vi "9941 Msg Received Event is null--error.vi"(8 "error in":errorcluster) -> (0 "error out":errorcluster, 2 "Error Code":i32)   [LabVIEW 2020, in "CANopen.lvlib" / "Response Matcher.lvclass"]
uses:
  Response Matcher.lvclass
  Response Matcher.lvclass/Response Matcher.ctl
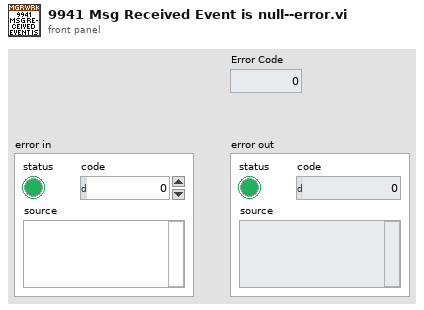
[diagram p1: front panel]
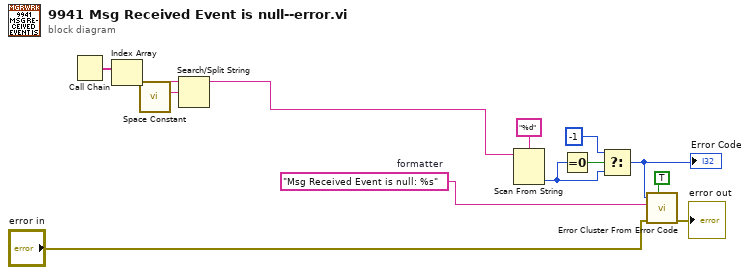
[diagram p0: block diagram]
diagram:
  w11 = "Msg Received Event is null: %s"  # formatter
  n1 = Call Chain() -> (call chain=w5:string[])
  n2 = Index Array(array=w5) -> (element=w9:string)  [unwired: 1 in]
  n3 = call <vilib>:"Space Constant.vi"() -> ("String"=w2:string)
  n4 = Search/Split String(string=w9, search string/char (-)=w2) -> (substring before match=w1:string)  [unwired: 1 in, 2 out]
  n5 = Scan From String(format string="%d", input string=w1) -> (output 1=w7:i32)  [unwired: 3 in, 3 out]
  n6 = Equal To 0?(x=w7) -> (x = 0?=w8:bool)
  n7 = Select(t=-1, s=w8, f=w7) -> (s? t:f=w4:i32)
  "Error Code" <- w4
  n8 = call <vilib>:"Error Cluster From Error Code.vi"("show call chain? (False)"=TRUE, "error in (no error)"="error in", "error message (\"\")"=w11, "error code (0)"=w4) -> ("error out"=→"error out":errorcluster)  [unwired: 5 in]
